vi "Pre Launch Init.vi"(11 "Nested in":refnum<class "Communicator Worker.lvclass">) -> (0 "error out":errorcluster, 3 "Nested out":refnum<class "Communicator Worker.lvclass">)   [LabVIEW 2019, in "Communicator Worker.lvlib" / "Communicator Worker.lvclass"]
doc: "(<B>Filename</B>: Actor Framework.lvlib:Actor.lvclass:Pre Launch Init.vi)\n\nDefines behavior that occurs after the Launch Nested Actor method is invoked but before the actor's Actor Core method begins running.\n\nBy default, this method does nothing. A descendant class may override it to define behavior."
uses:
  Communicator Worker.lvclass
  Communicator Worker.lvclass/Communicator Worker.ctl
  Interfaces/IMessage/IMessage.lvclass
  <vilib>/ActorFramework/Actor/Actor.lvclass
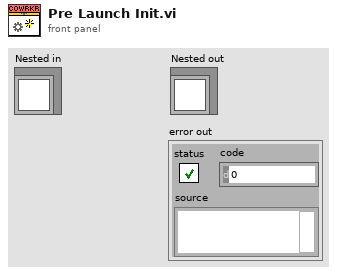
[diagram p1: front panel]
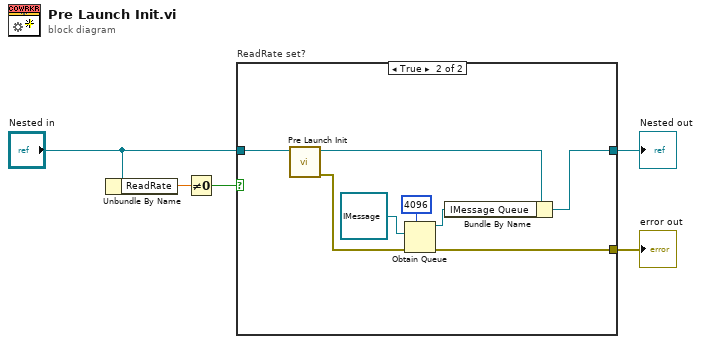
[diagram p0: block diagram]
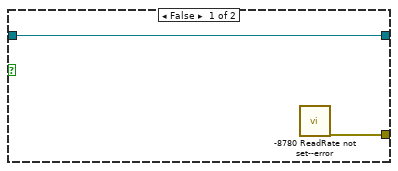
[diagram p2: hidden frame]
diagram:
  n1 = Unbundle By Name("Nested in") -> ("ReadRate"=w2:dbl)
  n2 = Not Equal To 0?(x=w2) -> (x != 0?=w1:bool)
  n3 = case "ReadRate set?" shown="True" w1 {
    tunnel: "Nested in" -> [w6 w13]
    tunnel: [w6 w15] -> w5
    tunnel: [w7 w14] -> w4
    frame False {
      n4 = call "-8780 ReadRate not set--error.vi"() -> ("error out"=w7:errorcluster)  [unwired: 11 in]
    }
    frame True {
      n5 = call-parent "Pre Launch Init.vi"("Actor in"=w13) -> ("error out"=w11:errorcluster, "Actor out"=w10:refnum<class "Communicator Worker.lvclass">)  [unwired: 9 in]
      n6 = Obtain Queue(max queue size (-1, unlimited)=4096, element data type=refnum<class "IMessage.lvclass"> refnum ("Communicate.lvlib:Message.lvclass"), error in (no error)=w11) -> (queue out=w9:refnum<queue>, error out=w14:errorcluster)  [unwired: 2 in, 1 out]
      n7 = Bundle By Name(cluster=w10, "IMessage Queue"=w9) -> (w15:refnum<class "Communicator Worker.lvclass">)
    }
  }
  "error out" <- w4
  "Nested out" <- w5
